vi "SCP_write_VS.vi"(8 "error_in":errorcluster, 9 "SCP_Cluster_in":T1, 10 "Ref":T2) -> (0 "error_out":errorcluster, 1 "SCP_Cluster_out":T1)   [LabVIEW 2023, in "Vires VTD Engine.lvlib"]
uses:
  Vires VTD Engine.lvlib
  Type/SCP_Cluster.ctl
  <vilib>/NI/NIVS Inline Async API/_Data Access Engine/Data Access Engine/Types/ReadWrite.DVR.ctl
  <vilib>/NI/NIVS Inline Async API/_Data Access Engine/Access Type Classes/ReadWrite/ReadWrite.lvclass
  <vilib>/NI/NIVS Inline Async API/_Data Access Engine/Access Type Classes/ReadWrite/ReadWrite.lvclass/ReadWrite.ctl
  <vilib>/NI/NIVS Inline Async API/_Data Access Engine/Data Access Engine/Methods/ReadWrite.Data.Write.vi
  <vilib>/NI/NIVS Inline Async API/_Data Access Engine/Access Type Classes/ReadWrite/ReadWrite.ProcessData.Write.vi
  <vilib>/NI/NIVS Inline Async API/_Data Access Engine/Access Type Classes/ReadWrite/ReadWrite.ProcessData.Buffer.vi
  <vilib>/NI/NIVS Inline Async API/_Data Access Engine/Access Type Classes/ReadWrite/ReadWrite.ProcessData.Commit.vi
  <vilib>/NI/NIVS Inline Async API/_Data Access Engine/Data Access Engine/Data Access Engine.lvclass
  SCP/SCP.lvlib
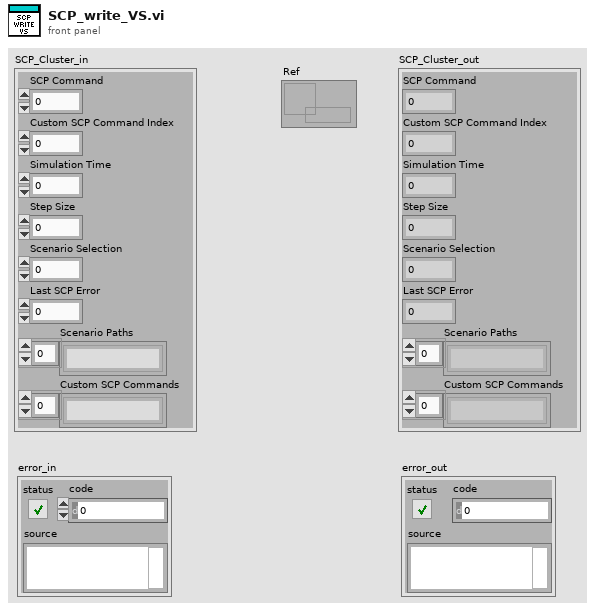
[diagram p1: front panel]
types:
  T1 = typedef "SCP.lvlib/SCP_Cluster.ctl" = cluster{"SCP Command ":i32, "Custom SCP Command Index":i32, "Simulation Time":i32, "Step Size":i32, "Scenario Selection":i32, "Last SCP Error":i32, "Scenario Paths":string[], "Custom SCP Commands":string[]}
  T2 = typedef "Data Access Engine.lvlib/Data Access Engine.lvclass/ReadWrite.DVR.ctl" = refnum<data-value>
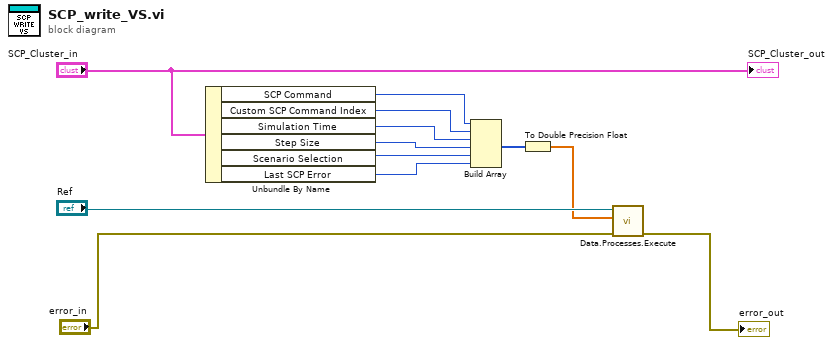
[diagram p0: block diagram]
diagram:
  n1 = Unbundle By Name("SCP_Cluster_in") -> ("SCP Command"=w8:i32, "Custom SCP Command Index"=w7:i32, "Simulation Time"=w6:i32, "Step Size"=w5:i32, "Scenario Selection"=w4:i32, "Last SCP Error"=w3:i32)
  n2 = Build Array(w8, w7, w6, w5, w4, w3) -> (w2:i32[])
  n3 = To Double Precision Float(number=w2) -> (double precision float=w1:dbl[])
  n4 = call-poly <vilib>:"Data.Processes.Execute.vi"("error in (no error)"="error_in", "Values"=w1, "Ref"="Ref") -> ("error out"=→"error_out":errorcluster)  [unwired: 8 in]
  "SCP_Cluster_out" <- "SCP_Cluster_in"
